vi "ejercicio 1.vi"() -> ()   [LabVIEW 2017]
panel:
  out "Computadoras total vendidas":i64
  out "Suma de filas":i64[](array[numeric])
  out "Suma de columnas":i64[](array[numeric])
  out "Vendedor que menos vendió":i64
  out "Zona que mas vendió":i64
  out "Arreglo 1":i64[][](array[numeric])
  # "Ejercicio 1\nEn un arreglo bidimensional de 3x4 que almacena la cantidad de computadoras\nvendidas por tres vendedores en cuatro zonasdiferentes. Genere numeros \naleatorios de 0 a 100 para llenar el arreglo. Se pide mostrar:\nLa zona que mas computadoras vendió\nEl vendedor que menos computadoras vendió.\nLa cantidad de computadoras vendidas por todos los vendedores en todas las zonas."
  # "Ejercicio 1"
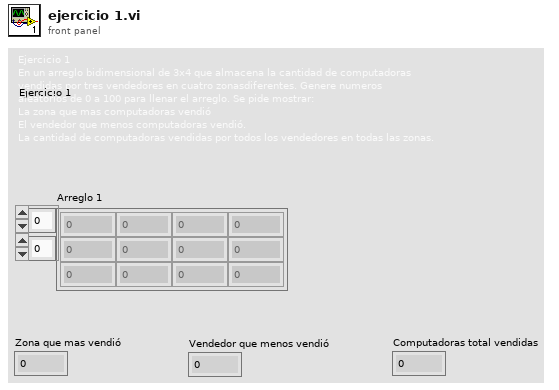
[diagram p1: front panel]
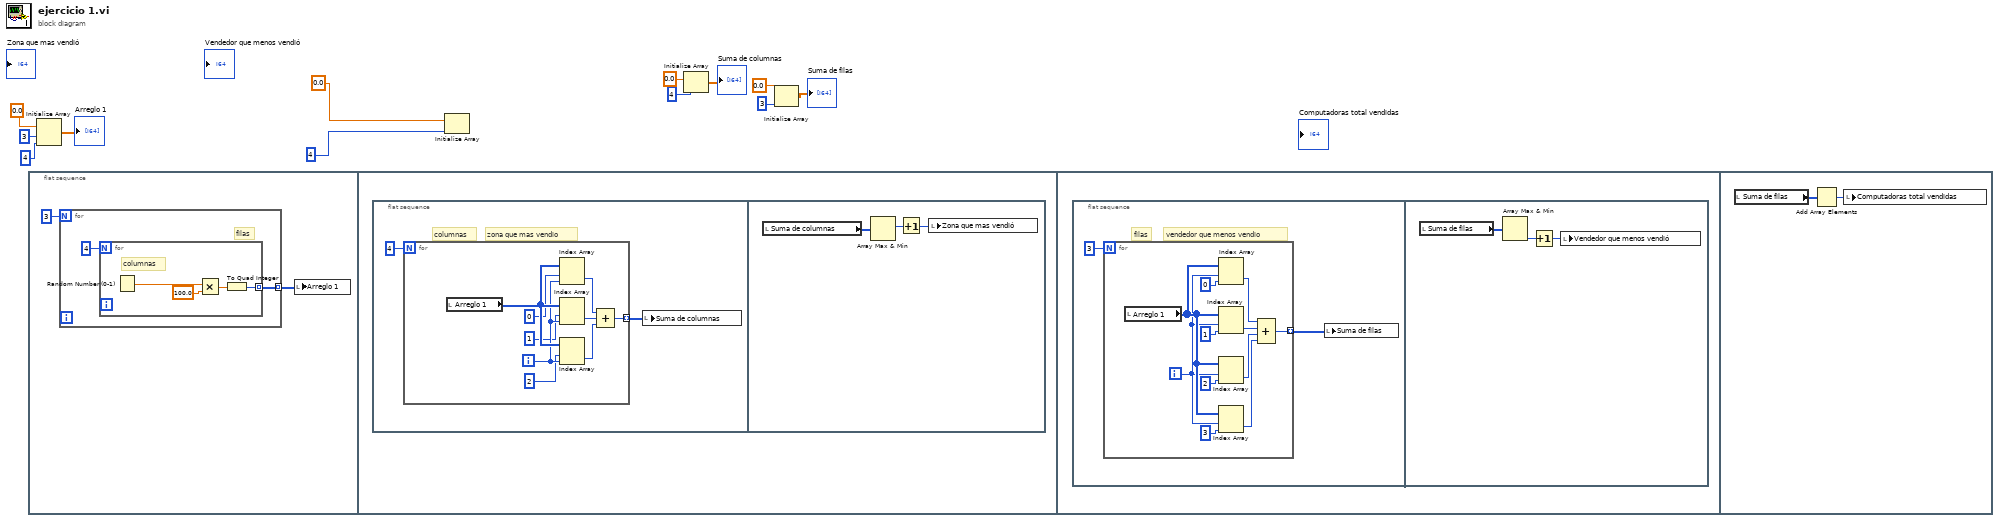
[diagram p0: block diagram]
diagram:
  n1 = flat-sequence {
    frame #0 {
      n2 = for {
        N: 3 -> [_]
        tunnel: [w15] -> w13 mode=indexing
        # "filas"
        n3 = for {
          N: 4 -> [_]
          tunnel: [w17] -> w15 mode=indexing
          # "columnas"
          n4 = Random Number (0-1)() -> (number: 0 to 1=w20:dbl)
          n5 = Multiply(x=w20, y=100.0) -> (x*y=w18:dbl)
          n6 = To Quad Integer(1:w18) -> (0:w17:i64)
        }
      }
      n7 = local write "Arreglo 1"(w13) -> ()
    }
    frame #1 {
      n8 = flat-sequence {
        frame #0 {
          # "zona que mas vendio"
          # "columnas"
          n9 = for {
            N: 4 -> [_]
            tunnel: [w24] -> w21 mode=indexing
            i -> [w30]
            n10 = local read "Arreglo 1"() -> (w31:i64[][])
            n11 = Index Array(array=w31, index (row)=0 ("disabled index (row)"), index (col)=w30) -> (element=w27:i64)
            n12 = Index Array(array=w31, index (row)=1 ("disabled index (row)"), index (col)=w30) -> (element=w26:i64)
            n13 = Index Array(array=w31, index (row)=2 ("disabled index (row)"), index (col)=w30) -> (element=w25:i64)
            n14 = Compound Arithmetic op=ADD(w27, w26, w25) -> (w24:i64)
          }
          n15 = local write "Suma de columnas"(w21) -> ()
        }
        frame #1 {
          n16 = local read "Suma de columnas"() -> (w34:i64[])
          n17 = Array Max & Min(array=w34) -> (max index (indices)=w33:i32)  [unwired: 3 out]
          n18 = Increment(x=w33) -> (x+1=w32:i32)
          n19 = local write "Zona que mas vendió"(w32) -> ()
        }
      }
    }
    frame #2 {
      n20 = flat-sequence {
        frame #0 {
          # "vendedor que menos vendio"
          # "filas"
          n21 = for {
            N: 3 -> [_]
            tunnel: [w43] -> w35 mode=indexing
            i -> [w41]
            n22 = local read "Arreglo 1"() -> (w42:i64[][])
            n23 = Index Array(array=w42, index (row)=w41, index (col)=0 ("disabled index (col)")) -> (element=w47:i64)
            n24 = Index Array(array=w42, index (row)=w41, index (col)=1 ("disabled index (col)")) -> (element=w46:i64)
            n25 = Index Array(array=w42, index (row)=w41, index (col)=2 ("disabled index (col)")) -> (element=w45:i64)
            n26 = Index Array(array=w42, index (row)=w41, index (col)=3 ("disabled index (col)")) -> (element=w44:i64)
            n27 = Compound Arithmetic op=ADD(w47, w46, w45, w44) -> (w43:i64)
          }
          n28 = local write "Suma de filas"(w35) -> ()
        }
        frame #1 {
          n29 = local read "Suma de filas"() -> (w50:i64[])
          n30 = Array Max & Min(array=w50) -> (min index (indices)=w49:i32)  [unwired: 3 out]
          n31 = Increment(x=w49) -> (x+1=w48:i32)
          n32 = local write "Vendedor que menos vendió"(w48) -> ()
        }
      }
    }
    frame #3 {
      n33 = local read "Suma de filas"() -> (w52:i64[])
      n34 = Add Array Elements(numeric array=w52) -> (sum=w51:i64)
      n35 = local write "Computadoras total vendidas"(w51) -> ()
    }
  }
  n36 = Initialize Array(0.0 ("element"), 3 ("dimension size"), 4 ("dimension size")) -> (→"Arreglo 1":dbl[][])
  n37 = Initialize Array(0.0 ("element"), 4 ("dimension size")) -> ()  [unwired: 1 out]
  n38 = Initialize Array(0.0 ("element"), 4 ("dimension size")) -> (→"Suma de columnas":dbl[])
  n39 = Initialize Array(0.0 ("element"), 3 ("dimension size")) -> (→"Suma de filas":dbl[])
